vi "setUp.vi"(8 "error in (no error)":errorcluster, 11 "Test Runner.Folder in":refnum<class "Test Runner.Folder.lvclass">) -> (0 "error out":errorcluster, 3 "Test Runner.Folder out":refnum<class "Test Runner.Folder.lvclass">)   [LabVIEW 2013, in "Caraya.lvlib" / "Test Runner.Folder.lvclass"]
uses:
  Test Runner.Folder.lvclass
  Test Runner/Test Runner.lvclass
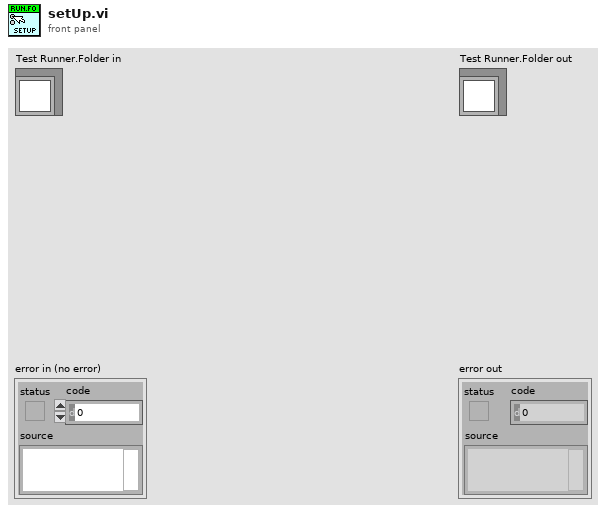
[diagram p1: front panel]
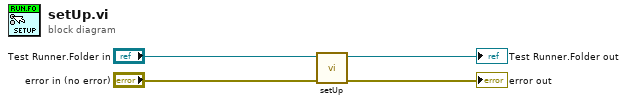
[diagram p0: block diagram]
diagram:
  n1 = call-parent "setUp.vi"("error in (no error)"="error in (no error)", "Test Runner in"="Test Runner.Folder in") -> ("error out"=→"error out":errorcluster, "Test Runner out"=→"Test Runner.Folder out":refnum<class "Test Runner.Folder.lvclass">)  [unwired: 8 in]
